vi "Begin.vi"(8 "error in":errorcluster) -> (0 "error out":errorcluster)   [LabVIEW 2016]
doc: "Called before other user functions, this VI is expected to open initial I/O refnums, load in file data, and do all program initialization. Notice that the <B>error out</B> terminal is simply used for data flow. Wiring it to other structures or subVIs ensures that this VI runs first."
uses:
  <vilib>/Rock Robotics/SystemInterfaces/DIO/FPGA_DIOPWMChannel.ctl
  <vilib>/Rock Robotics/WPI/SafetyOutput/WPI_SafetyOutputConfigMenu.ctl
  <vilib>/Rock Robotics/WPI/DriverStation/WPI_DriverStationRobotMode2.ctl
  <vilib>/Rock Robotics/WPI/Joystick/WPI_JoystickDeviceEnum.ctl
  <vilib>/Rock Robotics/SystemInterfaces/spilib/spi_bus.ctl
  <vilib>/Rock Robotics/WPI/Relay/WPI_RelayValue.ctl
  <vilib>/Rock Robotics/SystemInterfaces/DIO/FPGA_DIORelayChannel.ctl
  Robot Global Data.vi
  <vilib>/Rock Robotics/Network Tables/NT Write String Array.vi
  <vilib>/Rock Robotics/WPI/RobotDrive/WPI_RobotDriveOpen4MotorWithVictorSP.vi
  <vilib>/Rock Robotics/WPI/MotorControl/WPI_MotorControlOpen VictorSP.vi
  <vilib>/Rock Robotics/WPI/Gyro/WPI_GyroXRS450_SPI_Open.vi
  Global Current Values.vi
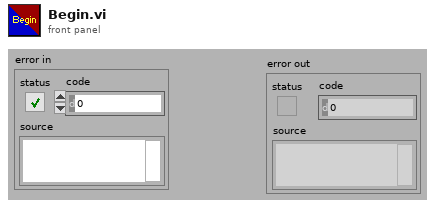
[diagram p1: front panel]
types:
  T1 = typedef "FPGA_DIOPWMChannel.ctl" = enum8{"PWM 0", "PWM 1", "PWM 2", "PWM 3", "PWM 4", "PWM 5", "PWM 6", "PWM 7", "PWM 8", "PWM 9", "PWM MXP 0", "PWM MXP 1", "PWM MXP 2", "PWM MXP 3", "PWM MXP 4", "PWM MXP 5", "PWM MXP 6", "PWM MXP 7", "PWM MXP 8", "PWM MXP 9", "Invalid"}
  T2 = typedef "FPGA_DIORelayChannel.ctl" = enum8{"Relay 0", "Relay 1", "Relay 2", "Relay 3", "Invalid"}
  T3 = typedef "WPI_RelayValue.ctl" = enum16{"Off", "On", "Forward", "Reverse"}
  T4 = typedef "spi_bus.ctl" = enum16{"SPI On-Board, CS0", "SPI On-Board, CS1", "SPI On-Board, CS2", "SPI On-Board, CS3", "SPI MXP", "Invalid"}
  T5 = typedef "WPI_JoystickDeviceEnum.ctl" = enum16{"USB 0", "USB 1", "USB 2", "USB 3", "USB 4", "USB 5"}
  T6 = typedef "WPI_DriverStationRobotMode2.ctl" = enum16{"Autonomous Disabled", "Autonomous Enabled", "Teleop Disabled", "Teleop Enabled", "Disconnected", "Finish", "Test Disabled", "Test Enabled", "Emergency Stopped"}
  T7 = typedef "WPI_SafetyOutputConfigMenu.ctl" = enum16{"Enable", "Disable"}
  T8 = typedef "WPI_MotorControlDeviceRef.ctl" = cluster{"DeviceStatus":errorcluster, "Type":T9, "PWM":cluster{"PWM Channel":T1, "DeadBand":T10}, "CAN":cluster{"Device Number":u8, "SetOutput VI Ref":variant, "GetOutput VI Ref":variant, "Enable VI Ref":variant, "Disable VI Ref":variant, "Data":variant}, "Invert":bool}
  T9 = typedef "WPI_MotorControlType.ctl" = enum16{"PWM", "CAN"}
  T10 = typedef "WPI_PWMDeadband.ctl" = cluster{"Name":string, "maxPositivePwm":i32, "minPositivePwm":i32, "centerPwm":i32, "maxNegativePwm":i32, "minNegativePwm":i32, "angularRange":u16}
  T11 = typedef "WPI_GyroDevRef.ctl" = cluster{"DevStatus":errorcluster, "Analog Channel":T12, "Offset":dbl, "Gain (VoltsPerDegree/Second)":dbl, "Gyro Type":enum16{"Analog", "XRS450"}, "Handle":i32, "SPI Bus":T4, "Device Found":bool, "Sample Rate":dbl, "Calibrate On Open":bool}
  T12 = typedef "FPGA_AIChannel.ctl" = enum8{"AI 0", "AI 1", "AI 2", "AI 3", "AI MXP 0", "AI MXP 1", "AI MXP 2", "AI MXP 3", "Invalid"}
  T13 = typedef "WPI_JoystickDevRef.ctl" = cluster{"Device":T5}
  T14 = typedef "WPI_RelayDevRef.ctl" = cluster{"DevStatus":errorcluster, "Relay Channel":T2, "Relay Direction":T15}
  T15 = typedef "WPI_RelayDirection.ctl" = enum16{"Both directions", "Forward only", "Reverse only"}
  T16 = typedef "WPI_RobotDriveDevRef.ctl" = cluster{"DevStatus":errorcluster, "Motors[]":T8[], "Square Inputs":bool, "Max Output":dbl}
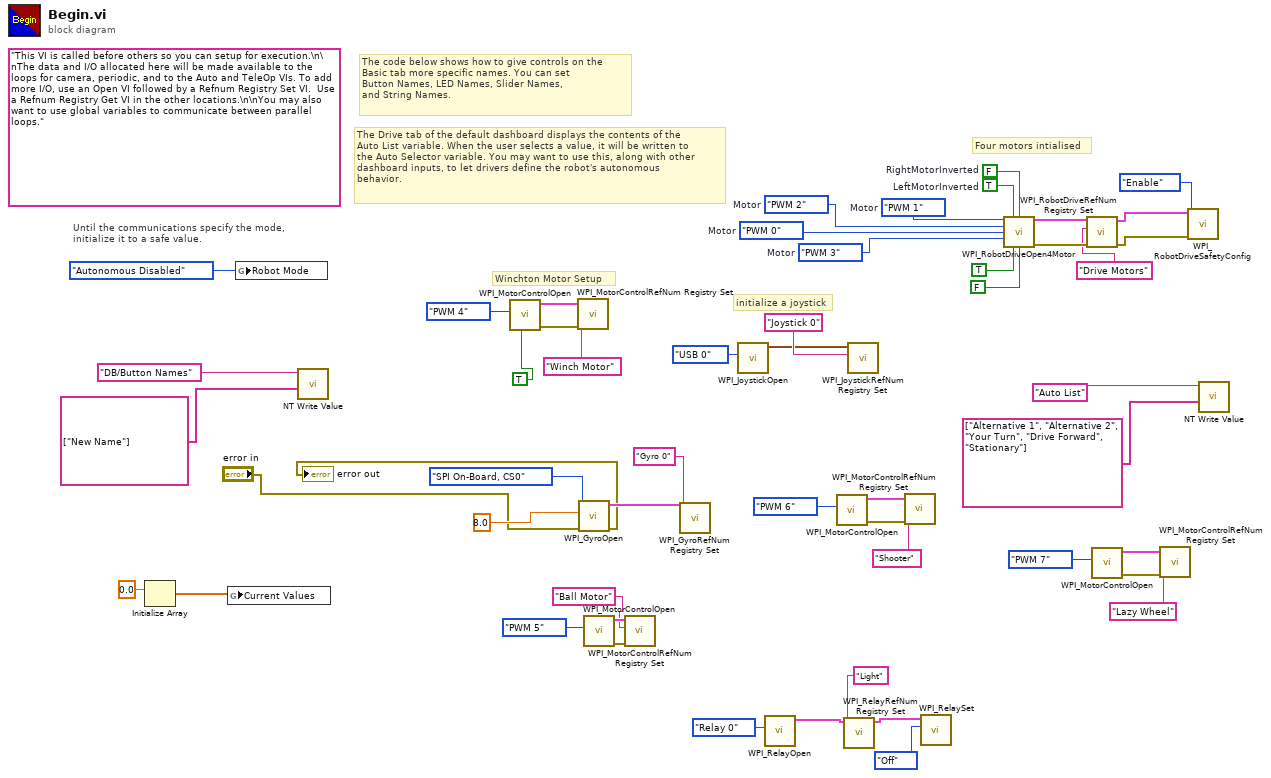
[diagram p0: block diagram]
diagram:
  w37 = FPGA_DIOPWMChannel."PWM 2"  # Motor
  w38 = FPGA_DIOPWMChannel."PWM 0"  # Motor
  (unwired) "This VI is called before others so you can setup for execution.\n\nThe data and I/O allocated here will be made available to the loops for camera, periodic, and to the Auto and TeleOp VIs. To add more I/O, use an Open VI followed by a Refnum Registry Set VI.  Use a Refnum Registry Get VI in the other locations.\n\nYou may also want to use global variables to communicate between parallel loops."
  w36 = FPGA_DIOPWMChannel."PWM 3"  # Motor
  w39 = FPGA_DIOPWMChannel."PWM 1"  # Motor
  w51 = TRUE  # LeftMotorInverted
  w52 = FALSE  # RightMotorInverted
  # "Winchton Motor Setup"
  # "The Drive tab of the default dashboard displays the contents of the\nAuto List variable. When the user selects a value, it will be written to\nthe Auto Selector variable. You may want to use this, along with other\ndashboard inputs, to let drivers define the robot's autonomous\nbehavior."
  # "The code below shows how to give controls on the\nBasic tab more specific names. You can set\nButton Names, LED Names, Slider Names,\nand String Names."
  # "initialize a joystick"
  # "Until the communications specify the mode,\ninitialize it to a safe value."
  # "Four motors intialised"
  n1 = Initialize Array(0.0 ("element")) -> (w18:dbl[])  [unwired: 1 in]
  n2 = global write "Global Current Values.vi" "Current Values"(w18) -> ()
  n3 = global write "Robot Global Data.vi" "Robot Mode"(WPI_DriverStationRobotMode2."Autonomous Disabled" ("Robot Mode")) -> ()
  n4 = call-poly <vilib>:"NT Write Value.vi"("String Array"=string[] ["New Name"], "Name"="DB/Button Names") -> ()  [unwired: 9 in, 1 out]
  n5 = call-poly <vilib>:"WPI_MotorControlOpen.vi"("Invert"=TRUE, "PWM Channel"=FPGA_DIOPWMChannel."PWM 4") -> ("error out"=w32:errorcluster, "MotorControlDeviceRef"=w26:T8)  [unwired: 8 in]
  n6 = call <vilib>:"WPI_MotorControlRefNum Registry Set.vi"("error in (no error)"=w32, "refnum name"="Winch Motor", "MotorControlDevRef"=w26) -> ()  [unwired: 7 in, 2 out]
  n7 = call-poly <vilib>:"WPI_GyroOpen.vi"("error in"="error in", "Sample Rate (ms)"=8.0, "SPI Bus"=spi_bus."SPI On-Board, CS0") -> ("error out"=→"error out":errorcluster, "GyroDevRef"=w23:T11)  [unwired: 7 in]
  n8 = call-poly <vilib>:"WPI_MotorControlOpen.vi"("PWM Channel"=FPGA_DIOPWMChannel."PWM 5") -> ("error out"=w3:errorcluster, "MotorControlDeviceRef"=w4:T8)  [unwired: 9 in]
  n9 = call <vilib>:"WPI_MotorControlRefNum Registry Set.vi"("error in (no error)"=w3, "refnum name"="Ball Motor", "MotorControlDevRef"=w4) -> ()  [unwired: 7 in, 2 out]
  n10 = call <vilib>:"WPI_GyroRefNum Registry Set.vi"("refnum name"="Gyro 0", "GyroDevRef"=w23) -> ()  [unwired: 8 in, 2 out]
  n11 = call <vilib>:"WPI_JoystickOpen.vi"("JoystickDevice"=WPI_JoystickDeviceEnum."USB 0") -> ("JoystickDevRef"=w46:T13)  [unwired: 10 in]
  n12 = call <vilib>:"WPI_RelayOpen.vi"("Relay Channel"=FPGA_DIORelayChannel."Relay 0") -> ("RelayDevRef"=w17:T14)  [unwired: 9 in, 1 out]
  n13 = call-poly <vilib>:"WPI_MotorControlOpen.vi"("PWM Channel"=FPGA_DIOPWMChannel."PWM 6") -> ("error out"=w11:errorcluster, "MotorControlDeviceRef"=w10:T8)  [unwired: 9 in]
  n14 = call <vilib>:"WPI_RelayRefNum Registry Set.vi"("refnum name"="Light", "RelayDevRef"=w17) -> ("RelayDevRef"=w16:T14)  [unwired: 8 in, 1 out]
  n15 = call <vilib>:"WPI_JoystickRefNum Registry Set.vi"("refnum name"="Joystick 0", "JoystickDevRef"=w46) -> ()  [unwired: 8 in, 2 out]
  n16 = call <vilib>:"WPI_MotorControlRefNum Registry Set.vi"("error in (no error)"=w11, "refnum name"="Shooter", "MotorControlDevRef"=w10) -> ()  [unwired: 7 in, 2 out]
  n17 = call <vilib>:"WPI_RelaySet.vi"("RelayValue"=WPI_RelayValue."Off", "RelayDevRef"=w16) -> ()  [unwired: 8 in, 2 out]
  n18 = call-poly <vilib>:"WPI_RobotDriveOpen4Motor.vi"("Rear Left Motor"=w39, "Rear Left Motor Inverted"=w51, "Rear Right Motor Inverted"=w52, "Rear Right Motor"=w37, "Front Left Motor"=w38, "Front Right Motor"=w36, "Front Left Motor Inverted"=TRUE, "Front Right Motor Inverted"=FALSE) -> ("RobotDriveDevRef"=w50:T16, "error out"=w40:errorcluster)  [unwired: 6 in]
  n19 = call <vilib>:"WPI_RobotDriveRefNum Registry Set.vi"("error in (no error)"=w40, "refnum name"="Drive Motors", "RobotDriveDevRef"=w50) -> ("error out"=w28:errorcluster, "RobotDriveDevRef"=w27:T16)  [unwired: 1 in, 6 out]
  n20 = call-poly <vilib>:"WPI_MotorControlOpen.vi"("PWM Channel"=FPGA_DIOPWMChannel."PWM 7") -> ("error out"=w7:errorcluster, "MotorControlDeviceRef"=w6:T8)  [unwired: 9 in]
  n21 = call <vilib>:"WPI_MotorControlRefNum Registry Set.vi"("error in (no error)"=w7, "refnum name"="Lazy Wheel", "MotorControlDevRef"=w6) -> ()  [unwired: 7 in, 2 out]
  n22 = call <vilib>:"WPI_RobotDriveSafetyConfig.vi"("error in (no error)"=w28, "mode"=WPI_SafetyOutputConfigMenu."Enable", "RobotDriveDevRef"=w27) -> ()  [unwired: 7 in, 2 out]
  n23 = call-poly <vilib>:"NT Write Value.vi"("String Array"=string[] ["Alternative 1", "Alternative 2", "Your Turn", "Drive Forward", "Stationary"], "Name"="Auto List") -> ()  [unwired: 9 in, 1 out]
